vi "overrideStim.vi"(8 "error in (no error)":errorcluster, 10 "Lick":bool, 11 "Stimulus in":refnum<class "Stimulus.lvclass">) -> (0 "error out":errorcluster, 1 "Lick Override":bool, 2 "Override":bool, 3 "Stimulus out":refnum<class "Stimulus.lvclass">)   [LabVIEW 2014, in "Stimulus.lvclass"]
uses:
  Stimulus.lvclass
  Stimulus.lvclass/Stimulus.ctl
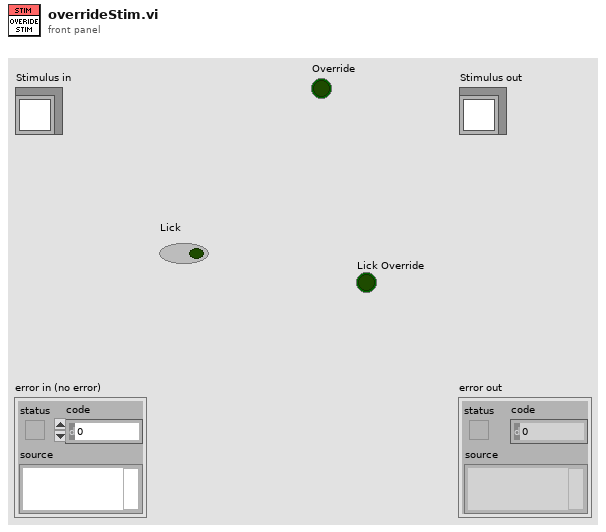
[diagram p1: front panel]
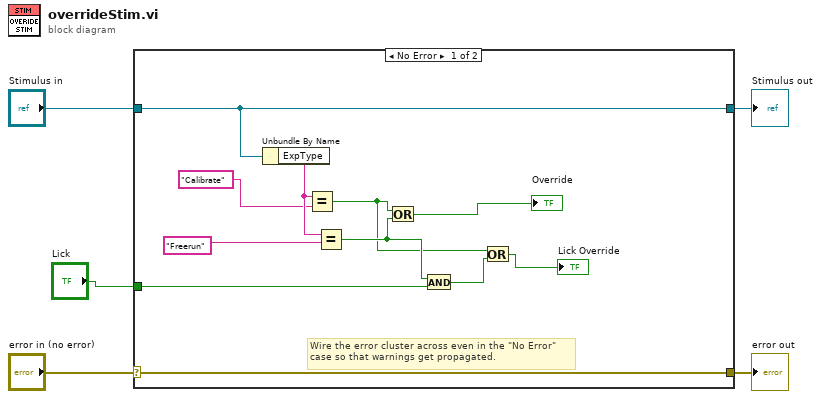
[diagram p0: block diagram]
diagram:
  n1 = case shown="No Error" "error in (no error)" {
    selector: "error in (no error)" -> [w16 w18]
    tunnel: [w16 w18] -> w4
    tunnel: [w15 w17] -> w2
    tunnel: "Stimulus in" -> [w15 w17]
    tunnel: "Lick" -> [w12 _]
    frame No Error {
      # "Wire the error cluster across even in the \"No Error\"\ncase so that warnings get propagated."
      n2 = Unbundle By Name(w15) -> ("ExpType"=w14:string)
      n3 = Equal?(x=w14, y="Calibrate" ("ExpType")) -> (x = y?=w8:bool)
      n4 = Equal?(x=w14, y="Freerun" ("ExpType")) -> (x = y?=w13:bool)
      n5 = Or(x=w8, y=w13) -> (x .or. y?=→"Override":bool)
      n6 = And(x=w13, y=w12) -> (x .and. y?=w11:bool)
      n7 = Or(x=w8, y=w11) -> (x .or. y?=→"Lick Override":bool)
    }
    frame Error {
    }
  }
  "error out" <- w4
  "Stimulus out" <- w2
